vi "AddContained.vi"(8 "error in (no error)":errorcluster, 9 "Item to contain":refnum<class "ILabVIEWItem.lvclass">, 11 "CLabVIEWItem in":refnum<class "CLabVIEWItem.lvclass">) -> (0 "error out":errorcluster, 1 "Relationship type":T1, 3 "CLabVIEWItem out":refnum<class "CLabVIEWItem.lvclass">)   [LabVIEW 2020, in "LabVIEWItem.lvlib" / "CLabVIEWItem.lvclass"]
uses:
  CLabVIEWItem.lvclass
  obj/Addons/LabVIEWObjectInterfaces.lvlibp/LabVIEWObjectInterfaces/ILabVIEWItem/ILabVIEWItem.lvclass
  CLabVIEWItem.lvclass/CLabVIEWItem.ctl
  obj/Addons/LabVIEWObjectInterfaces.lvlibp/LabVIEWObjectInterfaces/ILabVIEWItem/RelationshipType.ctl
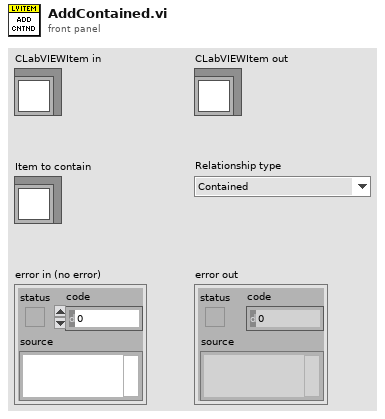
[diagram p1: front panel]
types:
  T1 = typedef "LabVIEWObjectInterfaces.lvlibp/ILabVIEWItem.lvclass/RelationshipType.ctl" = enum16{"Contained", "Dependency", "Parent", "Same item", "Related", "None"}
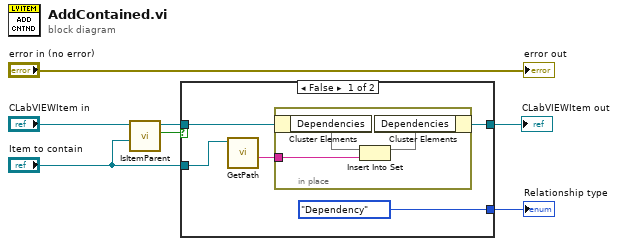
[diagram p0: block diagram]
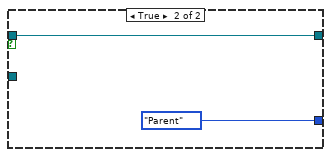
[diagram p2: hidden frame]
diagram:
  n1 = call-dynamic "IsItemParent.vi"("Item to compare"="Item to contain", "CLabVIEWItem in"="CLabVIEWItem in") -> ("Is parent?"=w2:bool, "CLabVIEWItem out"=w3:refnum<class "CLabVIEWItem.lvclass">)  [unwired: 7 in, 1 out]
  n2 = case shown="False" w2 {
    tunnel: w3 -> [w11 w17]
    tunnel: [w10 w17] -> w6
    tunnel: "Item to contain" -> [w9 _]
    tunnel: [RelationshipType."Dependency" ("Relationship type") RelationshipType."Parent" ("Relationship type")] -> w1
    frame False {
      n3 = call-dynamic "GetPath.vi"("ILabVIEWItem in"=w9) -> ("Path"=w12:string)  [unwired: 8 in, 2 out]
      n4 = in-place {
        in-place-border: w12 -> [w15]
        n5 = in-place-cluster #1(w11) -> ("Dependencies"=w14:set{string})
        n6 = Insert Into Set(10:w15, 11:w14) -> (3:w13:set{string})  [unwired: 1 out]
        n7 = in-place-cluster #1("Dependencies"=w13) -> (w10:refnum<class "CLabVIEWItem.lvclass">)
      }
    }
    frame True {
    }
  }
  "CLabVIEWItem out" <- w6
  "Relationship type" <- w1
  "error out" <- "error in (no error)"
